vi "Get_Quaternion.vi"(5 "Device Number":T1, 7 "Update":bool) -> (2 "Quaternion":T2)   [LabVIEW 2016]
doc: "This navX VI returns the quaternion of the navX."
uses:
  _TypeDefs/FRIC_navX_DeviceNumbersTypeDef.ctl
  _TypeDefs/Z900_navX_DeviceRegisters.ctl
  _Util/Z900_navX_Util_LittleEndian_to_BigEndian.vi
  _Internal/FRIC_navX_Get_Registry.vi
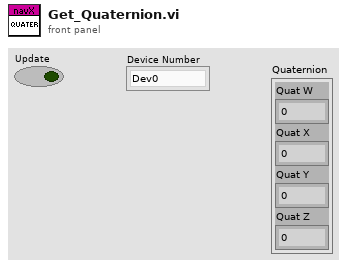
[diagram p1: front panel]
types:
  T1 = typedef "FRIC_navX_DeviceNumbersTypeDef.ctl" = enum16{"Dev0", "Dev1", "Dev2", "Dev3", "Dev4", "Dev5", "Dev6", "Dev7", "Dev8", "Dev9", "Dev10"}
  T2 = cluster{"Quat W":dbl, "Quat X":dbl, "Quat Y":dbl, "Quat Z":dbl}
  T3 = typedef "Z900_navX_DeviceRegisters.ctl" = u8
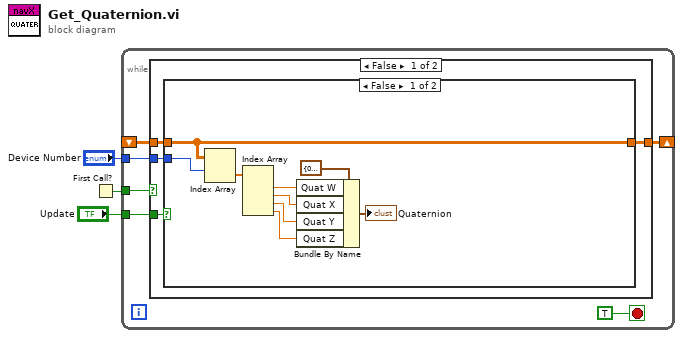
[diagram p0: block diagram]
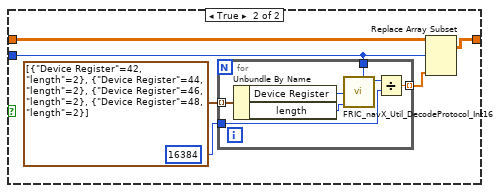
[diagram p2: hidden frame]
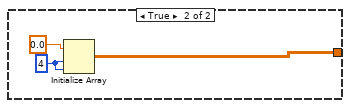
[diagram p3: hidden frame]
diagram:
  n1 = First Call?() -> (First Call?: T/F=w1:bool)
  n2 = while {
    shift-right: [w9] -> _
    shift-left: _ -> [w8]
    tunnel: "Update" -> [w6]
    tunnel: "Device Number" -> [w5]
    tunnel: w1 -> [w4]
    stop <- TRUE stop-if-true
    n3 = case shown="False" w4 {
      tunnel: [w13 w38] -> w9
      tunnel: w8 -> [w12 _]
      tunnel: w6 -> [w10 _]
      tunnel: w5 -> [w11 _]
      frame False {
        n4 = case shown="False" w10 {
          tunnel: [w21 w26] -> w13
          tunnel: w12 -> [w21 w27]
          tunnel: w11 -> [w22 w28]
          frame False {
            n5 = Index Array(array=w21, index (row)=w22) -> (element=w19:dbl[])  [unwired: 1 in]
            n6 = Index Array(array=w19) -> (element #1=w18:dbl, element #2=w17:dbl, element #3=w16:dbl, element #4=w15:dbl)  [unwired: 4 in]
            n7 = Bundle By Name(cluster=T2 {"Quat W"=0.0, "Quat X"=0.0, "Quat Y"=0.0, "Quat Z"=0.0}, "Quat W"=w18, "Quat X"=w17, "Quat Y"=w16, "Quat Z"=w15) -> (→"Quaternion":T2)
          }
          frame True {
            n8 = for {
              tunnel: cluster{"Device Register":T3, "length":i32}[] [{"Device Register"=42, "length"=2}, {"Device Register"=44, "length"=2}, {"Device Register"=46, "length"=2}, {"Device Register"=48, "length"=2}] ("Array") -> [w33] mode=indexing
              tunnel: w28 -> [w32]
              tunnel: u16 16384 ("y") -> [w30]
              tunnel: [w29] -> w23 mode=indexing
              n9 = Unbundle By Name(w33) -> ("Device Register"=w35:T3, "length"=w34:i32)
              n10 = call "FRIC_navX_Util_DecodeProtocol_Int16.vi"("Device Number"=w32, "length"=w34, "Device Register"=w35) -> ("Value"=w31:i16)  [unwired: 8 in]
              n11 = Divide(x=w31, y=w30) -> (x/y=w29:dbl)
            }
            n12 = Replace Array Subset(array=w27, new element=w23, index (row)=w28) -> (w26:dbl[][])  [unwired: 1 in]
          }
        }
      }
      frame True {
        w37 = 4 ("dimension size")
        n13 = Initialize Array(0.0, w37, w37) -> (w38:dbl[][])
      }
    }
  }
